vi "Categorize Timestamp Relativity NEW.vi"(1 "Newest Time Stamp":timestamp, 2 "Oldest Time Stamp":timestamp) -> (0 "Oldest Relative to Newest Time Stamp":string)   [LabVIEW 2011]
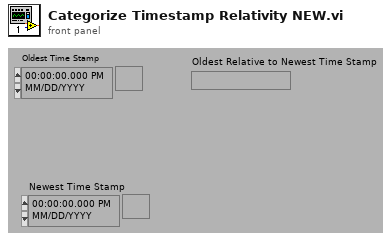
[diagram p1: front panel]
types:
  T1 = cluster{"second":i32, "minute":i32, "hour":i32, "day of month":i32, "month":i32, "year":i32, "day of week":i32, "day of year":i32, "is DST":i32}
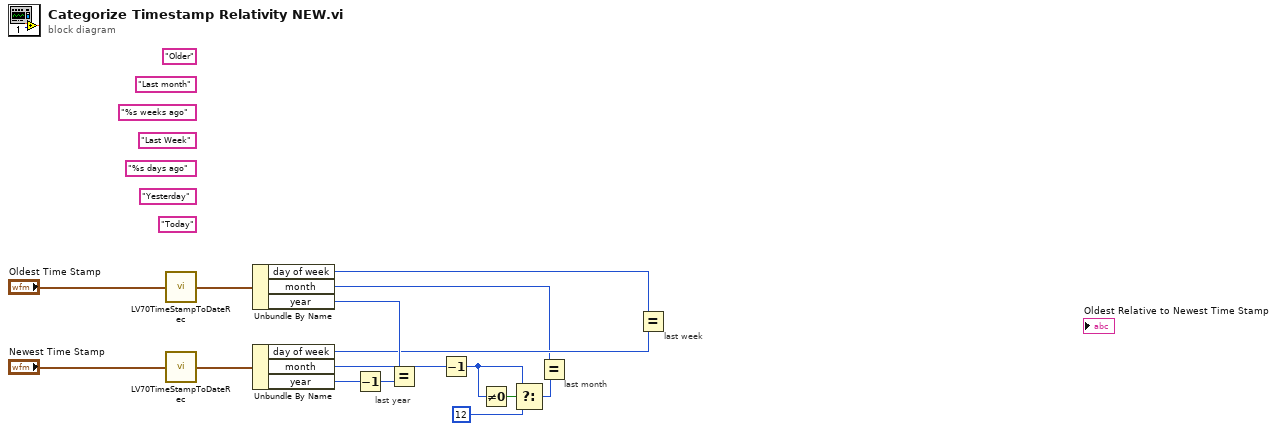
[diagram p0: block diagram]
diagram:
  (unwired) "%s weeks ago"
  (unwired) "Last Week"
  (unwired) "%s days ago"
  (unwired) "Last month"
  (unwired) "Older"
  (unwired) "Yesterday"
  (unwired) "Today"
  # "last week"
  # "last month"
  # "last year"
  n1 = call <vilib>:"LV70TimeStampToDateRec.vi"("time stamp"="Oldest Time Stamp") -> ("date time rec"=w15:T1)
  n2 = call <vilib>:"LV70TimeStampToDateRec.vi"("time stamp"="Newest Time Stamp") -> ("date time rec"=w12:T1)
  n3 = Unbundle By Name(w15) -> ("day of week"=w7:i32, "month"=w6:i32, "year"=w11:i32)
  n4 = Unbundle By Name(w12) -> ("day of week"=w8:i32, "month"=w4:i32, "year"=w10:i32)
  n5 = Decrement(x=w10) -> (x-1=w9:i32)
  n6 = Equal?(x=w11, y=w9) -> ()  [unwired: 1 out]
  n7 = Decrement(x=w4) -> (x-1=w3:i32)
  n8 = Not Equal To 0?(x=w3) -> (x != 0?=w5:bool)
  n9 = Select(t=w3, s=w5, f=12) -> (s? t:f=w2:i32)
  n10 = Equal?(x=w6, y=w2) -> ()  [unwired: 1 out]
  n11 = Equal?(x=w7, y=w8) -> ()  [unwired: 1 out]
